vi "c ctre phoenixpro get signal unit.vi"(8 "error in (no error)":errorcluster, 9 "max_size":u16, 10 "unit_c_string":string, 11 "spn":u16) -> (0 "error out":errorcluster, 2 "unit_c_string out":string, 3 "function return":i32)   [LabVIEW 2020, in "CTRE_PhoenixTools.lvlib"]
doc: "CTREXPORT int c_ctre_phoenixpro_get_signal_unit(\n uint16_t spn,\n char *unit_c_string, uint16_t max_size);"
uses:
  <userlib>/CTRE_PhoenixTools/CTRE_PhoenixTools.lvlib
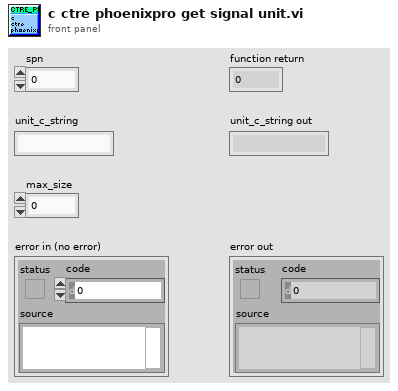
[diagram p1: front panel]
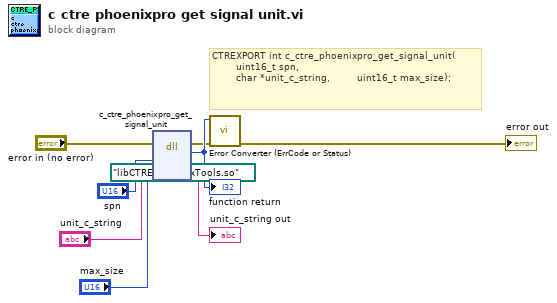
[diagram p0: block diagram]
diagram:
  # "CTREXPORT int c_ctre_phoenixpro_get_signal_unit(\n        uint16_t spn,\n        char *unit_c_string,         uint16_t max_size);"
  n1 = dll-call lib="?" fn="c_ctre_phoenixpro_get_signal_unit"(path in=path "libCTRE_PhoenixTools.so", error in="error in (no error)", "spn"="spn", "unit_c_string"="unit_c_string", "max_size"="max_size") -> (error out=w3:errorcluster, w9:i32, "unit_c_string"=→"unit_c_string out":string)  [unwired: 3 in, 1 out]
  "function return" <- w9
  n2 = call <userlib>:"Error Converter (ErrCode or Status).vi"("error in (no error)"=w3, "error code"=w9) -> ("error out"=→"error out":errorcluster)  [unwired: 9 in]
